vi "WBRT Close.vi"(8 "error in":errorcluster, 11 "WBRT State In":T1={"Encoders"={"Roll"=0.0, "Pitch"=0.0, "Yaw"=0.0, "Roll Trim"=0.0, "Pitch Trim"=0.0, "Yaw Trim"=0.0, "Roll Rate"=0.0, "Pitch Rate"=0.0, "Yaw Rate"=0.0}, "SPI Data"={"X-Gyro"=0.0, "Y-Gyro"=0.0, "Z-Gyro"=0.0, "X-Accel"=0.0, "Y-Accel"=0.0, "Z-Accel"=0.0}, "Camera"={"Numeric"=0.0}, "Filter Data"={"Filter Enabled?"=FALSE, "Filter Type"=enum."Equi-Ripple", "Pass Frequency"=1.0, "Stop Frequency (Equi-Ripple)"=0.45000000000000007, "Order"=0, "Ripple (dB)"=2.0}, "FPGA VI Reference"=refnum, "dt"=0.0, "Elapsed Time (msec)"=0, "Setpoints"={"Roll Setpoint (degrees)"=125.0, "Pitch Setpoint (degrees)"=125.0, "Yaw Setpoint (degrees)"=125.0}, "Commands"={"Left Command"=0.0, "Right Command"=0.0}, "Trajectory Data"=[], "Gains"={"Gain1"=0.0, "Gain2"=0.0, "Gain3"=0.0, "Gain4"=0.0, "Gain5"=0.0, "Gain6"=0.0, "Gain7"=0.0, "Gain8"=0.0, "Gain9"=0.0}, "Global Variables"={"Variable1"=[], "Variable2"=[], "Variable3"=[], "Variable4"=[]}, "Centroid"={"X Centroid"=0.0, "Y Centroid"=0.0}, "Error1"=0.0, "Error2"=0.0, "Error3"=0.0, "Error4"=0.0, "Recorded Data"=[], "Landing Factor"=0.0} {"Trajectory Data" format="%0.3f"; "Filter Data"."Stop Frequency (Equi-Ripple)" format="%0.3f"; "Filter Data"."Pass Frequency" format="%0.3f"}) -> (0 "error out":errorcluster)   [LabVIEW 2012]
doc: "Closes open references and zeros the outputs to the motor controllers.\n\nAuthor: Brandon Steele\n\nCopyright: Brigham Young University"
uses:
  Custom Controls/WBRT State.ctl
  Custom Controls/WBRT Encoders.ctl
  Custom Controls/WBRT SPI Data.ctl
  Custom Controls/WBRT Filter Data.ctl
  Custom Controls/WBRT Filter Type.ctl
  FPGA Samples/spi_single port_example/Host API/Controls/FPGA SPI_FPGA Ref.ctl
  Custom Controls/WBRT Setpoints.ctl
  Custom Controls/WBRT Commands.ctl
  Custom Controls/WBRT Gains.ctl
  Custom Controls/WBRT Global Variables.ctl
  <vilib>/Utility/error.llb/Error Cluster From Error Code.vi
  <vilib>/rvi/errors/niLvFpgaAdjustHostInterfaceError.vi
  <vilib>/FPGAPlugInAG/cRIO-9111/niLvFpga_Close_cRIO-9111.vi
  <vilib>/rvi/interface/nirviReadWriteControl/nirviReadWriteControl.xnode
  FPGA Bitfiles/Whirlybird_FPGATarget_WhirlybirdFPGAMa_DBA2D843.lvbitx
  Whirlybird FPGA Main.vi
  <vilib>/rvi/interface/nirviCloseFPGA/nirviCloseFPGA.xnode
  NiFpgaLv.dll
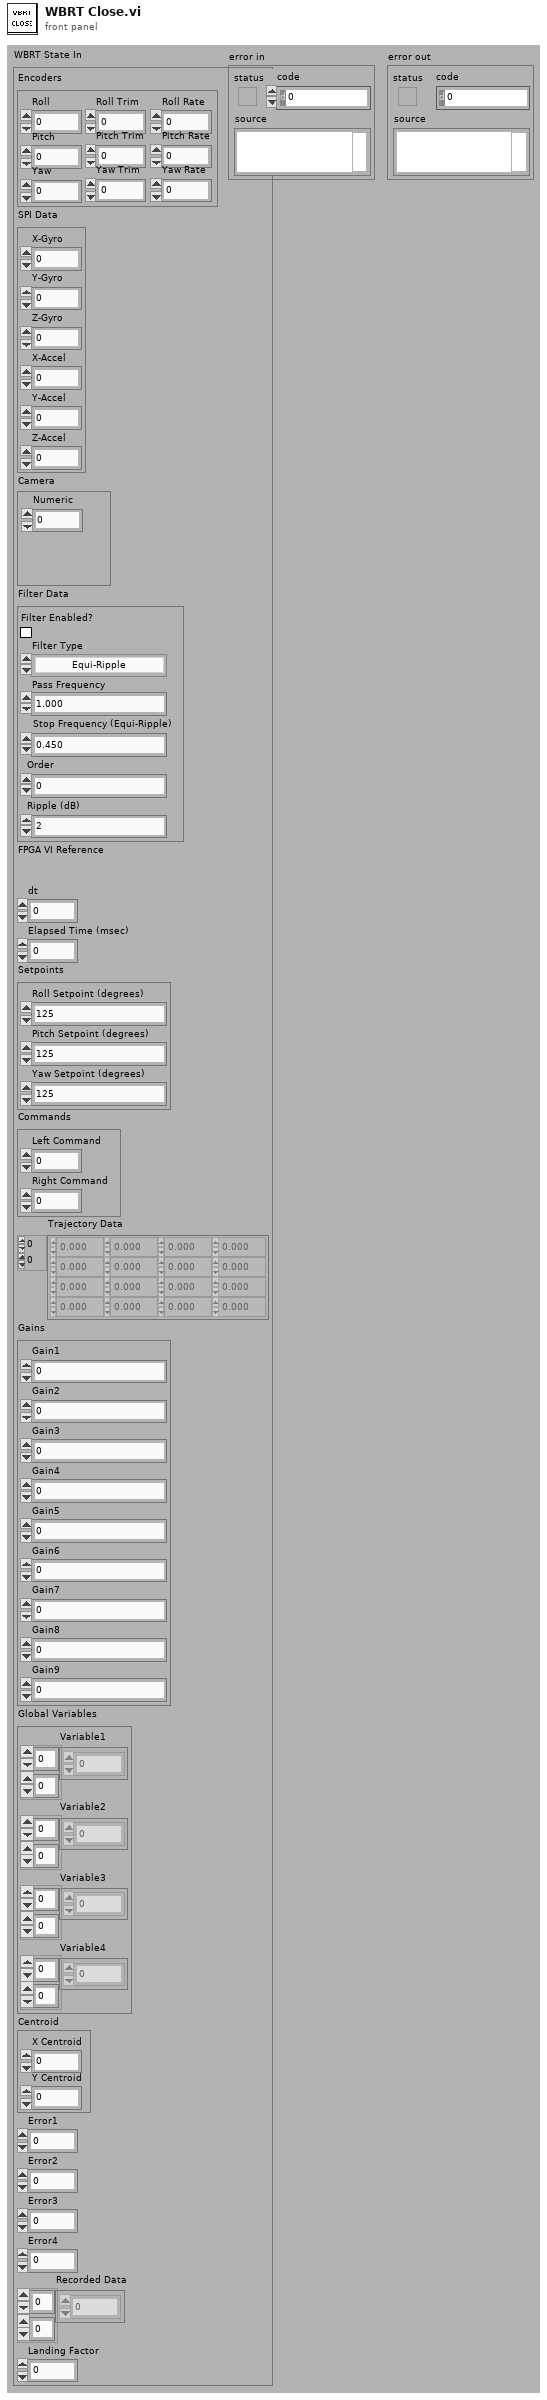
[diagram p1: front panel]
types:
  T1 = typedef "WBRT State.ctl" = cluster{"Encoders":T2, "SPI Data":T3, "Camera":cluster{"Numeric":dbl}, "Filter Data":T4, "FPGA VI Reference":T6, "dt":dbl, "Elapsed Time (msec)":u32, "Setpoints":T7, "Commands":T8, "Trajectory Data":dbl[][], "Gains":T9, "Global Variables":T10, "Centroid":cluster{"X Centroid":sgl, "Y Centroid":sgl}, "Error1":dbl, "Error2":dbl, "Error3":dbl, "Error4":dbl, "Recorded Data":dbl[][], "Landing Factor":dbl}
  T2 = typedef "WBRT Encoders.ctl" = cluster{"Roll":dbl, "Pitch":dbl, "Yaw":dbl, "Roll Trim":dbl, "Pitch Trim":dbl, "Yaw Trim":dbl, "Roll Rate":dbl, "Pitch Rate":dbl, "Yaw Rate":dbl}
  T3 = typedef "WBRT SPI Data.ctl" = cluster{"X-Gyro":dbl, "Y-Gyro":dbl, "Z-Gyro":dbl, "X-Accel":dbl, "Y-Accel":dbl, "Z-Accel":dbl}
  T4 = typedef "WBRT Filter Data.ctl" = cluster{"Filter Enabled?":bool, "Filter Type":T5, "Pass Frequency":dbl, "Stop Frequency (Equi-Ripple)":dbl, "Order":i32, "Ripple (dB)":dbl}
  T5 = typedef "WBRT Filter Type.ctl" = enum16{"Equi-Ripple", "Butterworth", "Chebyshev"}
  T6 = typedef "FPGA SPI_FPGA Ref.ctl" = refnum<k20>
  T7 = typedef "WBRT Setpoints.ctl" = cluster{"Roll Setpoint (degrees)":dbl, "Pitch Setpoint (degrees)":dbl, "Yaw Setpoint (degrees)":dbl}
  T8 = typedef "WBRT Commands.ctl" = cluster{"Left Command":dbl, "Right Command":dbl}
  T9 = typedef "WBRT Gains.ctl" = cluster{"Gain1":dbl, "Gain2":dbl, "Gain3":dbl, "Gain4":dbl, "Gain5":dbl, "Gain6":dbl, "Gain7":dbl, "Gain8":dbl, "Gain9":dbl}
  T10 = typedef "WBRT Global Variables.ctl" = cluster{"Variable1":dbl[][], "Variable2":dbl[][], "Variable3":dbl[][], "Variable4":dbl[][]}
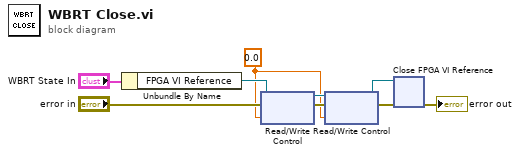
[diagram p0: block diagram]
diagram:
  w1 = 0.0 ("CommandA")
  n1 = Unbundle By Name("WBRT State In") -> ("FPGA VI Reference"=w6:T6)
  n2 = xnode "Read/Write Control"("FPGA VI Reference In"=w6, "error in"="error in", "MC2"=w1) -> ("FPGA VI Reference Out"=w8:T6, "error out"=w7:errorcluster)
  n3 = xnode "Read/Write Control"("FPGA VI Reference In"=w8, "error in"=w7, "MC1"=w1) -> ("FPGA VI Reference Out"=w2:T6, "error out"=w3:errorcluster)
  n4 = xnode "Close FPGA VI Reference"("FPGA VI Reference In"=w2, "error in"=w3) -> ("error out"=→"error out":errorcluster)
